vi "UpdateStateWithRef.vi"(0 "XRef":T8, 1 "Old State":T7, 2 "Version":T5) -> (14 "Is Good?":T4, 15 "Reply":T2, 16 "State Out":T1)   [LabVIEW 2012, in "ArrayDimension.xnode"]
doc: "This ability VI is called to perform mutation on an older version of an XNode. If a more recent version of an XNode's library exists, it will be called and let you mutate the old XNode's state appropriately to ensure compatibility with the newer XNode. If you want to report a warning on load of a VI containing an xnode that has its state updated, you can use the reply \"IssueWarning <Custom Load Warning goes here>\". Note that most LV load warnings begin with \"- \", so you will probably want to make yours conform to this standard. The load warning will only be issued if the state is successfully updated.\n\nDefault behavior: None.\n\nThis ability does not provide UI and OS messages are not handled."
uses:
  ArrayDimension.xnode
  <vilib>/XNodeSupport/XNodeXNodeRef.ctl
  <vilib>/XNodeSupport/XNodeVariant.ctl
  <vilib>/XNodeSupport/XNodeVersion.ctl
  <vilib>/XNodeSupport/XNodeUShort.ctl
  <vilib>/XNodeSupport/XNodeBool.ctl
  <vilib>/XNodeSupport/XNodeStringArray.ctl
  <vilib>/XNodeSupport/XNodeString.ctl
  State.ctl
  <vilib>/XNodeSupport/NI_XNodeSupport.lvlib
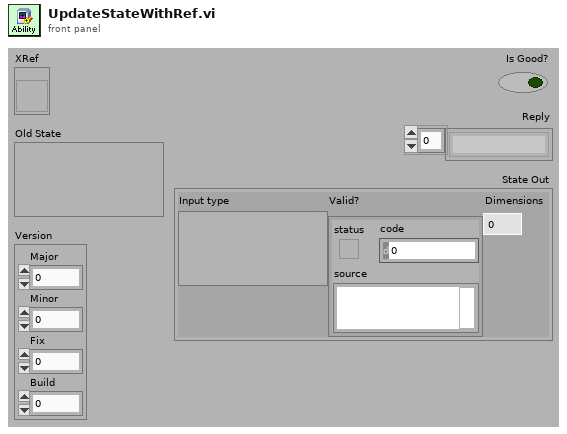
[diagram p1: front panel]
types:
  T1 = typedef "ArrayDimension.xnode/State.ctl" = cluster{"Input type":variant, "Valid?":errorcluster, "Dimensions":i32}
  T2 = typedef "NI_XNodeSupport.lvlib/XNodeStringArray.ctl" = T3[]
  T3 = typedef "NI_XNodeSupport.lvlib/XNodeString.ctl" = string
  T4 = typedef "NI_XNodeSupport.lvlib/XNodeBool.ctl" = bool
  T5 = typedef "NI_XNodeSupport.lvlib/XNodeVersion.ctl" = cluster{"Major":T6, "Minor":T6, "Fix":T6, "Build":T6}
  T6 = typedef "NI_XNodeSupport.lvlib/XNodeUShort.ctl" = u16
  T7 = typedef "NI_XNodeSupport.lvlib/XNodeVariant.ctl" = variant
  T8 = typedef "NI_XNodeSupport.lvlib/XNodeXNodeRef.ctl" = refnum<vi>
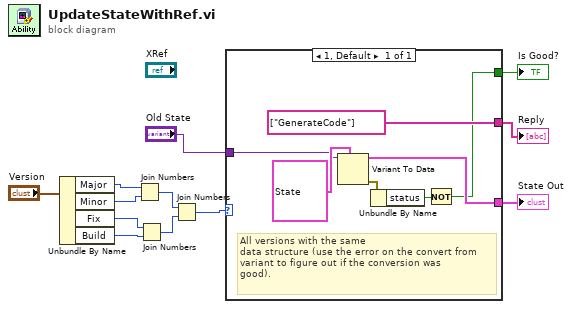
[diagram p0: block diagram]
diagram:
  n1 = Unbundle By Name("Version") -> ("Major"=w11:T6, "Minor"=w10:T6, "Fix"=w9:T6, "Build"=w8:T6)
  n2 = Join Numbers(hi=w11, lo=w10) -> ((hi.lo)=w7:u32)
  n3 = Join Numbers(hi=w9, lo=w8) -> ((hi.lo)=w6:u32)
  n4 = Join Numbers(hi=w7, lo=w6) -> ((hi.lo)=w5:u64)
  n5 = case shown="1, Default" w5 {
    tunnel: [w13] -> w4
    tunnel: [T2 ["GenerateCode"] ("Reply")] -> w3
    tunnel: "Old State" -> [w17]
    tunnel: [w16] -> w1
    frame 1, Default {
      # "All versions with the same\ndata structure (use the error on the convert from\nvariant to figure out if the conversion was\ngood)."
      n6 = Variant To Data(type=T1 {"Input type"=variant, "Valid?"={"status"=FALSE, "code"=0, "source"=""}, "Dimensions"=0} ("State"), Variant=w17) -> (data=w16:T1, error out=w15:errorcluster)  [unwired: 1 in]
      n7 = Unbundle By Name(w15) -> ("status"=w14:bool)
      n8 = Not(x=w14) -> (.not. x?=w13:bool)
    }
  }
  "Is Good?" <- w4
  "Reply" <- w3
  "State Out" <- w1
